vi "SAC-Read ASTFs.vi"(2 "State":T1, 7 "filestem":string, 11 "error in (no error)":errorcluster) -> (6 "IR":cluster{"offset":dbl, "dx":dbl, "Y":dbl[]}, 13 "phase":cluster{dbl, "dx":dbl, "Y":dbl[]}, 14 "mag":cluster{dbl, "dx":dbl, "Y":dbl[]}, 15 "error out":errorcluster)   [LabVIEW 2020]
uses:
  Typedefs/SAC-State.ctl
  Utility VIs/Conversion VIs/Create Waveform Cluster (1D).vi
  <vilib>/Analysis/NI_AALPro.lvlib
panel:
  out "error out":errorcluster
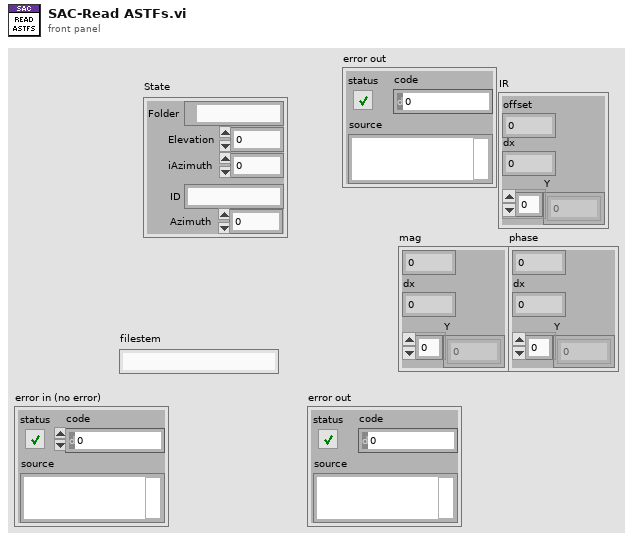
[diagram p1: front panel]
types:
  T1 = typedef "SAC-State.ctl" = cluster{"Folder":path, "Elevation":dbl, "iAzimuth":i32, "ID":string, "Azimuth":dbl}
  T2 = typedef "HRTF-filt Cluster.ctl" = cluster{"Type":string, "Fs":dbl, "a":dbl[], "b":dbl[], "window":i32, "Length_ms":dbl, "Center_ms":dbl}
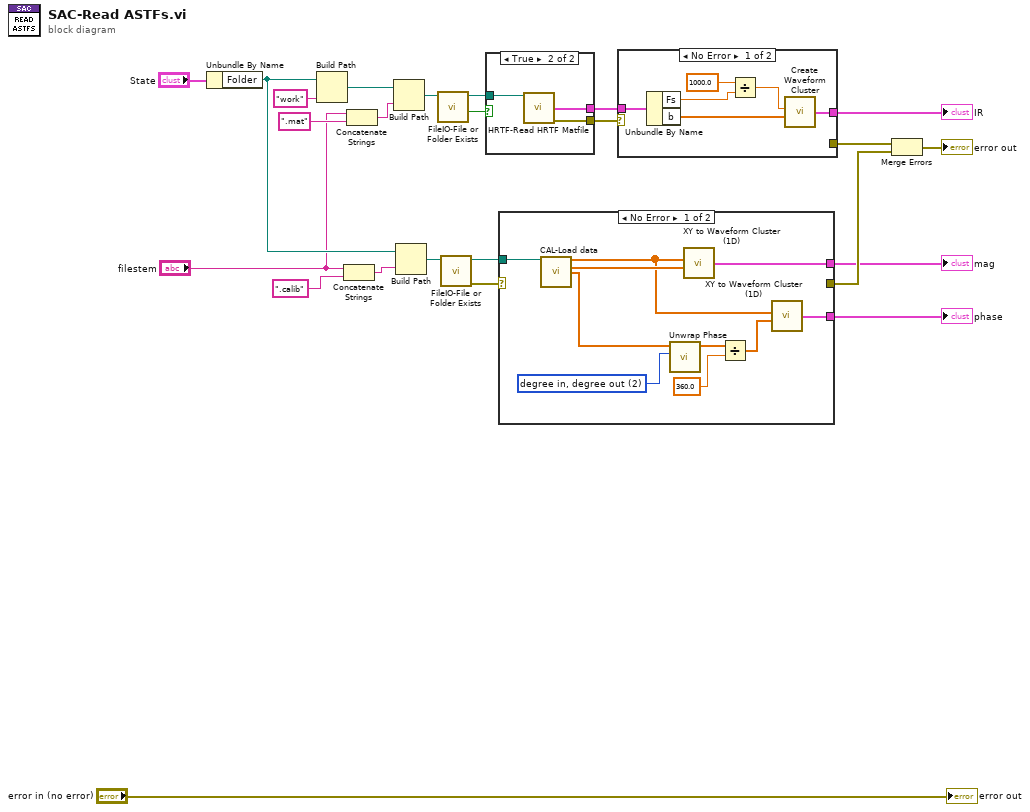
[diagram p0: block diagram]
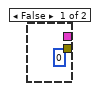
[diagram p2: hidden frame]
diagram:
  n1 = Unbundle By Name("State") -> ("Folder"=w12:path)
  n2 = Build Path(base path=w12, name or relative path="work") -> (appended path=w15:path)
  n3 = Concatenate Strings("filestem", ".calib" ("format string")) -> (w10:string)
  n4 = Concatenate Strings("filestem", ".mat" ("format string")) -> (w13:string)
  n5 = Build Path(base path=w15, name or relative path=w13) -> (appended path=w19:path)
  n6 = Build Path(base path=w12, name or relative path=w10) -> (appended path=w8:path)
  n7 = call "FileIO-File or Folder Exists.vi"("path"=w19) -> ("Exists?"=w17:bool, "dup path"=w18:path)  [unwired: 7 in, 2 out]
  n8 = call "FileIO-File or Folder Exists.vi"("path"=w8) -> ("error out"=w5:errorcluster, "dup path"=w7:path)  [unwired: 7 in, 2 out]
  n9 = case shown="True" w17 {
    tunnel: w18 -> [_ w27]
    tunnel: [_ w25] -> w21
    tunnel: [_ w26] -> w22
    frame False {
      (unwired) 0
    }
    frame True {
      n10 = call "HRTF-Read HRTF Matfile.vi"("path"=w27) -> ("filt"=w25:T2, "error out"=w26:errorcluster)  [unwired: 13 in]
    }
  }
  n11 = case shown="No Error" w5 {
    selector: w5 -> [_ w38]
    tunnel: w7 -> [w37 _]
    tunnel: [_ w38] -> w3
    tunnel: [w31 _] -> w2
    tunnel: [w28 _] -> w1
    frame No Error {
      w36 = 2 items=["radian in, radian out", "radian in, degree out", "degree in, degree out", "degree in, radian out"] ("phase unit")
      n12 = call "CAL-Load data.vi"("user path"=w37) -> ("Frequency (Hz)"=w30:dbl[], "Mag"=w32:dbl[], "Phase"=w34:dbl[])  [unwired: 7 in, 5 out]
      n13 = call <vilib>:"Unwrap Phase.vi"("phase unit"=w36, "Phase"=w34) -> ("Unwrapped Phase"=w33:dbl[])  [unwired: 8 in, 1 out]
      n14 = call "XY to Waveform Cluster (1D).vi"("X"=w30, "Y"=w32) -> ("waveform cluster"=w31:cluster{dbl, "dx":dbl, "Y":dbl[]})  [unwired: 3 in]
      n15 = Divide(x=w33, y=360.0) -> (x/y=w29:dbl[])
      n16 = call "XY to Waveform Cluster (1D).vi"("X"=w30, "Y"=w29) -> ("waveform cluster"=w28:cluster{dbl, "dx":dbl, "Y":dbl[]})  [unwired: 3 in]
    }
    frame Error {
    }
  }
  "mag" <- w2
  "phase" <- w1
  n17 = case shown="No Error" w22 {
    selector: w22 -> [_ w45]
    tunnel: w21 -> [w44 _]
    tunnel: [_ w45] -> w20
    tunnel: [w39 _] -> w6
    frame No Error {
      n18 = Unbundle By Name(w44) -> ("Fs"=w41:dbl, "b"=w40:dbl[])
      n19 = Divide(x=1000.0, y=w41) -> (x/y=w43:dbl)
      n20 = call-poly "Create Waveform Cluster.vi"("dx"=w43, "Y"=w40) -> ("waveform cluster"=w39:cluster{dbl, "dx":dbl, "Y":dbl[]})  [unwired: 3 in]
    }
    frame Error {
    }
  }
  "IR" <- w6
  n21 = Merge Errors(w20, w3) -> (→"error out":errorcluster)
  "error out" <- "error in (no error)"
